vi "rsscope_core_global.vi"() -> ()   [LabVIEW 2018] (continued)
the advanced jitter measurement subsystem (option K133). You can set a separate scale for the symbol rate and symbol duration basic jitter components. You can also set one scale for all other jitter components."}, {"Level"=6, "Class Only"=FALSE, "Identifier"="RSSCOPE_ATTR_ADVANCED_JITTER_RESULTS_SCALING_MAX_NUM_OF_BINS", "Descriptive Name"="Advanced Jitter Results Scaling Max Num Of Bins", "Data Type"=0, "Command"="ADVJ{AdvJitterMeas}:RES:VERT:HBIN", "Access"=2, "Range Table"="RsScope_rngAdvancedJitterHistogramBins", "Read Callback"="", "Write Callback"="", "Supported Models"="", "Instrument Options"="K133|K134", "Flags"=0, "Help"="Sets the number of bins, the number of data intervals, of the histogram.\n\nAvailable Repeated Capabilities:\nAdvJitterMeas: JA1, JA2\r\n\nRemote-control command(s):\nADVJitter<m>:RESult:VERTical:HBINs"}, {"Level"=6, "Class Only"=FALSE, "Identifier"="RSSCOPE_ATTR_ADVANCED_JITTER_RESULTS_CONTINUOUS_AUTO_SCALE_ENABLED", "Descriptive Name"="Advanced Jitter Results Continuous Auto Scale Enabled", "Data Type"=3, "Command"="ADVJ{AdvJitterMeas}:RES:VERT:CONT", "Access"=2, "Range Table"="", "Read Callback"="", "Write Callback"="", "Supported Models"="", "Instrument Options"="K133|K134", "Flags"=0, "Help"="If enabled, the measurement scale is set automatically. If disabled you can manually set a RSSCOPE_ATTR_ADVANCED_JITTER_RESULTS_COMPONENT_SCALE and a RSSCOPE_ATTR_ADVANCED_JITTER_RESULTS_COMPONENT_OFFSET.\n\nAvailable Repeated Capabilities:\nAdvJitterMeas: JA1, JA2\r\n\nRemote-control command(s):\nADVJitter<m>:RESult:VERTical:CONTinuous"}, {"Level"=6, "Class Only"=FALSE, "Identifier"="RSSCOPE_ATTR_ADVANCED_JITTER_RESULTS_BASIC_JITTER_CONTINUOUS_AUTO_SCALE_ENABLED", "Descriptive Name"="Advanced Jitter Results Basic Jitter Continuous Auto Scale Enabled", "Data Type"=3, "Command"="ADVJ{AdvJitterMeas}:RES:VERT:BHC", "Access"=2, "Range Table"="", "Read Callback"="", "Write Callback"="", "Supported Models"="", "Instrument Options"="K133|K134", "Flags"=0, "Help"="If enabled, the measurement scale of the basic jitter measurement histogram and track is set automatically. If disabled you can manually set a scale (RSSCOPE_ATTR_ADVANCED_JITTER_RESULTS_COMPONENT_SCALE) and an offset (RSSCOPE_ATTR_ADVANCED_JITTER_RESULTS_COMPONENT_OFFSET).\n\nAvailable Repeated Capabilities:\nAdvJitterMeas: JA1, JA2\r\n\nRemote-control command(s):\nADVJitter<m>:RESult:VERTical:BHContinuous"}, {"Level"=6, "Class Only"=FALSE, "Identifier"="RSSCOPE_ATTR_ADVANCED_JITTER_RESULTS_NOISE_CONTINUOUS_AUTO_SCALE_ENABLED", "Descriptive Name"="Advanced Jitter Results Noise Continuous Auto Scale Enabled", "Data Type"=3, "Command"="ADVJ{AdvJitterMeas}:RES:VERT:NHC", "Access"=2, "Range Table"="", "Read Callback"="", "Write Callback"="", "Supported Models"="", "Instrument Options"="K133|K134", "Flags"=0, "Help"="If enabled, the measurement scale of the noise histogram and track is set automatically. If disabled you can manually set a scale (RSSCOPE_ATTR_ADVANCED_JITTER_RESULTS_COMPONENT_SCALE) and an offset (RSSCOPE_ATTR_ADVANCED_JITTER_RESULTS_COMPONENT_OFFSET).\n\nAvailable Repeated Capabilities:\nAdvJitterMeas: JA1, JA2\r\n\nRemote-control command(s):\nADVJitter<m>:RESult:VERTical:NHContinuous"}, {"Level"=6, "Class Only"=FALSE, "Identifier"="RSSCOPE_ATTR_ADVANCED_JITTER_RESULTS_JITTER_SPECTRUM_CONTINUOUS_AUTO_SCALE_ENABLED", "Descriptive Name"="Advanced Jitter Results Jitter Spectrum Continuous Auto Scale Enabled", "Data Type"=3, "Command"="ADVJ{AdvJitterMeas}:RES:VERT:JSC", "Access"=2, "Range Table"="", "Read Callback"="", "Write Callback"="", "Supported Models"="", "Instrument Options"="K133|K134", "Flags"=0, "Help"="If enabled, the measurement scale of the jitter spectrum is set automatically. If disabled you can manually set a scale (RSSCOPE_ATTR_ADVANCED_JITTER_RESULTS_COMPONENT_SCALE) and an offset (RSSCOPE_ATTR_ADVANCED_JITTER_RESULTS_COMPONENT_OFFSET).\n\nAvailable Repeated Capabilities:\nAdvJitterMeas: JA1, JA2\r\n\nRemote-control command(s):\nADVJitter<m>:RESult:VERTical:JSContinuous"}, {"Level"=6, "Class Only"=FALSE, "Identifier"="RSSCOPE_ATTR_ADVANCED_JITTER_RESULTS_NOISE_SPECTRUM_CONTINUOUS_AUTO_SCALE_ENABLED", "Descriptive Name"="Advanced Jitter Results Noise Spectrum Continuous Auto Scale Enabled", "Data Type"=3, "Command"="ADVJ{AdvJitterMeas}:RES:VERT:NSC", "Access"=2, "Range Table"="", "Read Callback"="", "Write Callback"="", "Supported Models"="", "Instrument Options"="K133|K134", "Flags"=0, "Help"="If enabled, the measurement scale for the noise spectrum is set automatically. If disabled you can manually set a scale (RSSCOPE_ATTR_ADVANCED_JITTER_RESULTS_COMPONENT_SCALE) and an offset (RSSCOPE_ATTR_ADVANCED_JITTER_RESULTS_COMPONENT_OFFSET).\n\nAvailable Repeated Capabilities:\nAdvJitterMeas: JA1, JA2\r\n\nRemote-control command(s):\nADVJitter<m>:RESult:VERTical:NSContinuous"}, {"Level"=6, "Class Only"=FALSE, "Identifier"="RSSCOPE_ATTR_ADVANCED_JITTER_RESULTS_SCALING_MEASUREMENT_TYPE", "Descriptive Name"="Advanced Jitter Results Scaling Measurement Type", "Data Type"=0, "Command"="ADVJ{AdvJitterMeas}:RES:VERT:BMTY", "Access"=2, "Range Table"="RsScope_rngAdvancedJitterScalingMeasurement", "Read Callback"="", "Write Callback"="", "Supported Models"="", "Instrument Options"="K133|K134", "Flags"=0, "Help"="Selects the basic measurement type to apply the vertical scale to.\n\nAvailable Repeated Capabilities:\nAdvJitterMeas: JA1, JA2\r\n\nRemote-control command(s):\nADVJitter<m>:RESult:VERTical:BMTYpe"}, {"Level"=5, "Class Only"=TRUE, "Identifier"="", "Descriptive Name"="Periodic", "Data Type"=0, "Command"="", "Access"=0, "Range Table"="", "Read Callback"="", "Write Callback"="", "Supported Models"="", "Instrument Options"="", "Flags"=0, "Help"="This class contains results specific to periodic components in the advanced jitter measurement subsystem (option K133)"}, {"Level"=6, "Class Only"=FALSE, "Identifier"="RSSCOPE_ATTR_ADVANCED_JITTER_RESULTS_PERIODIC_COMPONENT_COUNT", "Descriptive Name"="Advanced Jitter Results Periodic Component Count", "Data Type"=0, "Command"="ADVJ{AdvJitterMeas}:RES:PER:COUN?", "Access"=0, "Range Table"="", "Read Callback"="", "Write Callback"="", "Supported Models"="", "Instrument Options"="K133|K134", "Flags"=0, "Help"="Returns the number of periodic components.\n\nAvailable Repeated Capabilities:\nAdvJitterMeas: JA1, JA2\r\n\nRemote-control command(s):\nADVJitter<m>:RESult:PERiodic<n>:COUNt?"}, {"Level"=6, "Class Only"=FALSE, "Identifier"="RSSCOPE_ATTR_ADVANCED_JITTER_RESULTS_PERIODIC_COMPONENT_FREQUENCY", "Descriptive Name"="Advanced Jitter Results Periodic Component Frequency", "Data Type"=5, "Command"="ADVJ{AdvJitterMeas}:RES:PER{AdvJitterPeriodicComponent}?", "Access"=0, "Range Table"="RsScope_rngAdvancedJitterPeriodicFrequency", "Read Callback"="", "Write Callback"="", "Supported Models"="", "Instrument Options"="K133|K134", "Flags"=0, "Help"="Returns the frequency of the selected periodic component.\n\nAvailable Repeated Capabilities:\nAdvJitterMeas: JA1, JA2\r\nAdvJitterPeriodicComponent: Periodic1, Periodic2, Periodic3, Periodic4, Periodic5, Periodic6, Periodic7, Periodic8, Periodic9, Periodic10\r\n\nRemote-control command(s):\nADVJitter<m>:RESult:PERiodic<n>[:FREQuency]?"}, {"Level"=6, "Class Only"=FALSE, "Identifier"="RSSCOPE_ATTR_ADVANCED_JITTER_RESULTS_PERIODIC_COMPONENT_VALUE", "Descriptive Name"="Advanced Jitter Results Periodic Component Value", "Data Type"=1, "Command"="ADVJ{AdvJitterMeas}:RES:PER{AdvJitterPeriodicComponent}:VAL?", "Access"=0, "Range Table"="", "Read Callback"="", "Write Callback"="", "Supported Models"="", "Instrument Options"="K133|K134", "Flags"=0, "Help"="Returns the value of the selected periodic component.\n\nAvailable Repeated Capabilities:\nAdvJitterMeas: JA1, JA2\r\nAdvJitterPeriodicComponent: Periodic1, Periodic2, Periodic3, Periodic4, Periodic5, Periodic6, Periodic7, Periodic8, Periodic9, Periodic10\r\n\nRemote-control command(s):\nADVJitter<m>:RESult:PERiodic<n>:VALue?"}, {"Level"=6, "Class Only"=FALSE, "Identifier"="RSSCOPE_ATTR_ADVANCED_JITTER_RESULTS_PERIODIC_COMPONENT_DIRECTION", "Descriptive Name"="Advanced Jitter Results Periodic Component Direction", "Data Type"=0, "Command"="ADVJ{AdvJitterMeas}:RES:PER{AdvJitterPeriodicComponent}:DIR?", "Access"=0, "Range Table"="RsScope_rngAdvancedJitterPeriodicDirection", "Read Callback"="", "Write Callback"="", "Supported Models"="", "Instrument Options"="K133|K134", "Flags"=0, "Help"="Returns the direction of the selected periodic component.\n\nAvailable Repeated Capabilities:\nAdvJitterMeas: JA1, JA2\r\nAdvJitterPeriodicComponent: Periodic1, Periodic2, Periodic3, Periodic4, Periodic5, Periodic6, Periodic7, Periodic8, Periodic9, Periodic10\r\n\nRemote-control command(s):\nADVJitter<m>:RESult:PERiodic<n>:DIRection?"}, {"Level"=2, "Class Only"=TRUE, "Identifier"="", "Descriptive Name"="Eye Jitter Measurements", "Data Type"=0, "Command"="", "Access"=0, "Range Table"="", "Read Callback"="", "Write Callback"="", "Supported Models"="", "Instrument Options"="", "Flags"=0, "Help"="The eye diagram is a significant means of visualizing jitter and allows you to analyze the reasons for it. Characteristic values can be identified in the eye diagram, and by creating histograms of the eye diagram, important jitter parameters can be determined. In the R&S RTO, the eye diagram is automatically set up for jitter measurements."}, {"Level"=3, "Class Only"=FALSE, "Identifier"="RSSCOPE_ATTR_EYE_MAIN_MEASUREMENT", "Descriptive Name"="Eye Jitter Main Measurement", "Data Type"=0, "Command"="MEAS{Measurement}:MAIN", "Access"=2, "Range Table"="rsscope_rngEyeJitterMeasurementType", "Read Callback"="", "Write Callback"="", "Supported Models"="", "Instrument Options"="", "Flags"=0, "Help"="Defines or queries the main measurement. This measurement is the one referred to if the measurement waveform is used as a source for math calculations. The main measurement type must belong to the same category as the other types assigned to the same measurement waveform, if there are any.\n\nAvailable Repeated Capabilities:\nMeasurement: Meas1, Meas2, Meas3, Meas4, Meas5, Meas6, Meas7, Meas8, Meas9, Meas10\r\n\nRemote-control command(s):\nMEASurement<m>:MAIN"}, {"Level"=3, "Class Only"=FALSE, "Identifier"="RSSCOPE_ATTR_EYE_JITTER_AUTOSCALE", "Descriptive Name"="Eye Jitter Autoscale", "Data Type"=4, "Command"="MEAS{Measurement}:EYEJ:AUT", "Access"=1, "Range Table"="", "Read Callback"="", "Write Callback"="", "Supported Models"="", "Instrument Options"="", "Flags"=0, "Help"="Defines optimized settings to perform an eye diagram measurement for the selected source.\n\nAvailable Repeated Capabilities:\nMeasurement: Meas1, Meas2, Meas3, Meas4, Meas5, Meas6, Meas7, Meas8, Meas9, Meas10\r\n\nRemote-control command(s):\nMEASurement<m>:EYEJitter:AUToscale"}, {"Level"=3, "Class Only"=TRUE, "Identifier"="", "Descriptive Name"="Eye Measurement Type", "Data Type"=0, "Command"="", "Access"=0, "Range Table"="", "Read Callback"="", "Write Callback"="", "Supported Models"="", "Instrument Options"="", "Flags"=0, "Help"="Selects Eye Measurement Type"}, {"Level"=4, "Class Only"=FALSE, "Identifier"="RSSCOPE_ATTR_EYE_LIMIT_CHECK", "Descriptive Name"="Eye Jitter Limit Check", "Data Type"=0, "Command"="MEAS{Measurement}:EYEJ:LCH{EyeMeasurementType}:VAL", "Access"=2, "Range Table"="rsscope_rngLimitCheck", "Read Callback"="", "Write Callback"="", "Supported Models"="", "Instrument Options"="", "Flags"=0, "Help"="Enables or disables limit checking for eye/jitter measurements in the specified measurement channel.\n\nAvailable Repeated Capabilities:\nMeasurement: Meas1, Meas2, Meas3, Meas4, Meas5, Meas6, Meas7, Meas8, Meas9, Meas10\r\nEyeMeasurementType: Eye1, Eye2, Eye3, Eye4, Eye5, Eye6, Eye7, Eye8, Eye9, Eye10, Eye11, Eye12, Eye13, Eye14, Eye15, Eye16, Eye17, Eye18, Eye19, Eye20, Eye21, Eye22, Eye23, Eye24, Eye25, Eye26, Eye27, Eye28, Eye29, Eye30\r\n\nRemote-control command(s):\nMEASurement<m>:EYEJitter:LCHeck<n>:VALid"}, {"Level"=4, "Class Only"=FALSE, "Identifier"="RSSCOPE_ATTR_EYE_JITTER_LOWER_LIMIT_VALUE", "Descriptive Name"="Eye Jitter Lower Limit Value", "Data Type"=1, "Command"="MEAS{Measurement}:EYEJ:LCH{EyeMeasurementType}:LOW:LIM", "Access"=2, "Range Table"="", "Read Callback"="", "Write Callback"="", "Supported Models"="", "Instrument Options"="", "Flags"=0, "Help"="Define the lower limit for the limit check.\n\nAvailable Repeated Capabilities:\nMeasurement: Meas1, Meas2, Meas3, Meas4, Meas5, Meas6, Meas7, Meas8, Meas9, Meas10\r\nEyeMeasurementType: Eye1, Eye2, Eye3, Eye4, Eye5, Eye6, Eye7, Eye8, Eye9, Eye10, Eye11, Eye12, Eye13, Eye14, Eye15, Eye16, Eye17, Eye18, Eye19, Eye20, Eye21, Eye22, Eye23, Eye24, Eye25, Eye26, Eye27, Eye28, Eye29, Eye30\r\n\nRemote-control command(s):\nMEASurement<m>:EYEJitter:LCHeck<n>:LOWer:LIMit"}, {"Level"=4, "Class Only"=FALSE, "Identifier"="RSSCOPE_ATTR_EYE_JITTER_UPPER_LIMIT_VALUE", "Descriptive Name"="Eye Jitter Upper Limit Value", "Data Type"=1, "Command"="MEAS{Measurement}:EYEJ:LCH{EyeMeasurementType}:UPP:LIM", "Access"=2, "Range Table"="", "Read Callback"="", "Write Callback"="", "Supported Models"="", "Instrument Options"="", "Flags"=0, "Help"="Define the upper limit for the limit check.\n\nAvailable Repeated Capabilities:\nMeasurement: Meas1, Meas2, Meas3, Meas4, Meas5, Meas6, Meas7, Meas8, Meas9, Meas10\r\nEyeMeasurementType: Eye1, Eye2, Eye3, Eye4, Eye5, Eye6, Eye7, Eye8, Eye9, Eye10, Eye11, Eye12, Eye13, Eye14, Eye15, Eye16, Eye17, Eye18, Eye19, Eye20, Eye21, Eye22, Eye23, Eye24, Eye25, Eye26, Eye27, Eye28, Eye29, Eye30\r\n\nRemote-control command(s):\nMEASurement<m>:EYEJitter:LCHeck<n>:UPPer:LIMit"}, {"Level"=4, "Class Only"=FALSE, "Identifier"="RSSCOPE_ATTR_EYE_JITTER_LOWER_LIMIT_MARGIN", "Descriptive Name"="Eye Jitter Lower Limit Margin", "Data Type"=1, "Command"="MEAS{Measurement}:EYEJ:LCH{EyeMeasurementType}:LOW:MARG", "Access"=2, "Range Table"="", "Read Callback"="", "Write Callback"="", "Supported Models"="", "Instrument Options"="", "Flags"=0, "Help"="Defines the lower margin for the limit check. Margins are not as strict as limits and must be within the valid value range.\n\nAvailable Repeated Capabilities:\nMeasurement: Meas1, Meas2, Meas3, Meas4, Meas5, Meas6, Meas7, Meas8, Meas9, Meas10\r\nEyeMeasurementType: Eye1, Eye2, Eye3, Eye4, Eye5, Eye6, Eye7, Eye8, Eye9, Eye10, Eye11, Eye12, Eye13, Eye14, Eye15, Eye16, Eye17, Eye18, Eye19, Eye20, Eye21, Eye22, Eye23, Eye24, Eye25, Eye26, Eye27, Eye28, Eye29, Eye30\r\n\nRemote-control command(s):\nMEASurement<m>:EYEJitter:LCHeck<n>:LOWer:MARGin"}, {"Level"=4, "Class Only"=FALSE, "Identifier"="RSSCOPE_ATTR_EYE_JITTER_UPPER_LIMIT_MARGIN", "Descriptive Name"="Eye Jitter Upper Limit Margin", "Data Type"=1, "Command"="MEAS{Measurement}:EYEJ:LCH{EyeMeasurementType}:UPP:MARG", "Access"=2, "Range Table"="", "Read Callback"="", "Write Callback"="", "Supported Models"="", "Instrument Options"="", "Flags"=0, "Help"="Defines the upper margin for the limit check. Margins are not as strict as limits and must be within the valid value range.\n\nAvailable Repeated Capabilities:\nMeasurement: Meas1, Meas2, Meas3, Meas4, Meas5, Meas6, Meas7, Meas8, Meas9, Meas10\r\nEyeMeasurementType: Eye1, Eye2, Eye3, Eye4, Eye5, Eye6, Eye7, Eye8, Eye9, Eye10, Eye11, Eye12, Eye13, Eye14, Eye15, Eye16, Eye17, Eye18, Eye19, Eye20, Eye21, Eye22, Eye23, Eye24, Eye25, Eye26, Eye27, Eye28, Eye29, Eye30\r\n\nRemote-control command(s):\nMEASurement<m>:EYEJitter:LCHeck<n>:UPPer:MARGin"}, {"Level"=2, "Class Only"=TRUE, "Identifier"="", "Descriptive Name"="Histograms", "Data Type"=0, "Command"="", "Access"=0, "Range Table"="", "Read Callback"="", "Write Callback"="", "Supported Models"="", "Instrument Options"="", "Flags"=0, "Help"="Histograms are used to plot density of data, i.e. to display graphically how often which signal values occur. In the R&S RTO, the histogram can be based on the input signal levels (amplitudes) or the time base in a time domain measurement, or on frequencies or frequency levels in a spectrum measurement.\nDepending on which data the histogram is based on, a vertical or horizontal histogram can be selected. A vertical, or amplitude, histogram displays horizontal bars across amplitude values. A horizontal or time/frequency histogram displays vertical bars over time/frequencies."}, {"Level"=3, "Class Only"=FALSE, "Identifier"="RSSCOPE_ATTR_HISTOGRAM_MAIN_MEASUREMENT", "Descriptive Name"="Histogram Main Measurement", "Data Type"=0, "Command"="MEAS{Measurement}:MAIN", "Access"=2, "Range Table"="rsscope_rngHistogramMeasurementType", "Read Callback"="", "Write Callback"="", "Supported Models"="", "Instrument Options"="", "Flags"=0, "Help"="Defines or queries the main measurement. This measurement is the one referred to if the measurement waveform is used as a source for math calculations. The main measurement type must belong to the same category as the other types assigned to the same measurement waveform, if there are any.\n\nAvailable Repeated Capabilities:\nMeasurement: Meas1, Meas2, Meas3, Meas4, Meas5, Meas6, Meas7, Meas8, Meas9, Meas10\r\n\nRemote-control command(s):\nMEASurement<m>:MAIN"}, {"Level"=3, "Class Only"=FALSE, "Identifier"="RSSCOPE_ATTR_HISTOGRAM_SELECT", "Descriptive Name"="Histogram Select", "Data Type"=2, "Command"="MEAS{Measurement}:HIST:SEL", "Access"=2, "Range Table"="", "Read Callback"="", "Write Callback"="", "Supported Models"="", "Instrument Options"="", "Flags"=0, "Help"="Selects the histogram on which the measurement is based.\n\nAvailable Repeated Capabilities:\nMeasurement: Meas1, Meas2, Meas3, Meas4, Meas5, Meas6, Meas7, Meas8, Meas9, Meas10\r\n\nRemote-control command(s):\nMEASurement<m>:HISTogram:SELect"}, {"Level"=3, "Class Only"=FALSE, "Identifier"="RSSCOPE_ATTR_HISTOGRAM_PROBABILITY_TYPE", "Descriptive Name"="Histogram Probability Type", "Data Type"=0, "Command"="MEAS{Measurement}:HIST:PROB:TYPE", "Access"=2, "Range Table"="rsscope_rngProbabilityType", "Read Callback"="", "Write Callback"="", "Supported Models"="", "Instrument Options"="", "Flags"=0, "Help"="Defines the marker reference in the probability domain.\n\nAvailable Repeated Capabilities:\nMeasurement: Meas1, Meas2, Meas3, Meas4, Meas5, Meas6, Meas7, Meas8, Meas9, Meas10\r\n\nRemote-control command(s):\nMEASurement<m>:HISTogram:PROBability:TYPE"}, {"Level"=3, "Class Only"=FALSE, "Identifier"="RSSCOPE_ATTR_HISTOGRAM_PROBABILITY_LIMIT", "Descriptive Name"="Histogram Probability Limit", "Data Type"=0, "Command"="MEAS{Measurement}:HIST:PROB:LIM", "Access"=2, "Range Table"="rsscope_rngPct", "Read Callback"="", "Write Callback"="", "Supported Models"="", "Instrument Options"="", "Flags"=0, "Help"="Defines a range around the probability marker.\n\nAvailable Repeated Capabilities:\nMeasurement: Meas1, Meas2, Meas3, Meas4, Meas5, Meas6, Meas7, Meas8, Meas9, Meas10\r\n\nRemote-control command(s):\nMEASurement<m>:HISTogram:PROBability:LIMit"}, {"Level"=3, "Class Only"=FALSE, "Identifier"="RSSCOPE_ATTR_REMOVE_HISTOGRAM", "Descriptive Name"="Remove Histogram", "Data Type"=2, "Command"="LAY:HIST:REM", "Access"=1, "Range Table"="", "Read Callback"="", "Write Callback"="", "Supported Models"="", "Instrument Options"="", "Flags"=0, "Help"="Removes the specified histogram.\n\nAvailable Repeated Capabilities:\nNone\n\nRemote-control command(s):\nLAYout:HISTogram:REMove"}, {"Level"=3, "Class Only"=FALSE, "Identifier"="RSSCOPE_ATTR_RESET_HISTOGRAM", "Descriptive Name"="Reset Histogram", "Data Type"=2, "Command"="LAY:HIST:RES", "Access"=1, "Range Table"="", "Read Callback"="", "Write Callback"="", "Supported Models"="", "Instrument Options"="", "Flags"=0, "Help"="Resets the values to begin a new histogram.\n\nAvailable Repeated Capabilities:\nNone\n\nRemote-control command(s):\nLAYout:HISTogram:RESet"}, {"Level"=3, "Class Only"=FALSE, "Identifier"="RSSCOPE_ATTR_HISTOGRAM_DISPLAY", "Descriptive Name"="Histogram Display", "Data Type"=3, "Command"="MEAS{Measurement}:DISP:HIST", "Access"=2, "Range Table"="", "Read Callback"="", "Write Callback"="", "Supported Models"="", "Instrument Options"="", "Flags"=0, "Help"="Displays a histogram for the source of the selected measurement.\n\nAvailable Repeated Capabilities:\nMeasurement: Meas1, Meas2, Meas3, Meas4, Meas5, Meas6, Meas7, Meas8, Meas9, Meas10\r\n\nRemote-control command(s):\nMEASurement<m>:DISPlay:HISTogram"}, {"Level"=3, "Class Only"=TRUE, "Identifier"="", "Descriptive Name"="Histogram Measurement Type", "Data Type"=0, "Command"="", "Access"=0, "Range Table"="", "Read Callback"="", "Write Callback"="", "Supported Models"="", "Instrument Options"="", "Flags"=0, "Help"="Selects Histogram Measurement Type"}, {"Level"=4, "Class Only"=FALSE, "Identifier"="RSSCOPE_ATTR_HISTOGRAM_LIMIT_CHECK", "Descriptive Name"="Histogram Limit Check", "Data Type"=0, "Command"="MEAS{Measurement}:HIST:LCH{HistogramMeasurementType}:VAL", "Access"=2, "Range Table"="rsscope_rngLimitCheck", "Read Callback"="", "Write Callback"="", "Supported Models"="", "Instrument Options"="", "Flags"=0, "Help"="Enables or disables limit checking for histogram measurements in the specified measurement channel.\n\nAvailable Repeated Capabilities:\nMeasurement: Meas1, Meas2, Meas3, Meas4, Meas5, Meas6, Meas7, Meas8, Meas9, Meas10\r\nHistogramMeasurementType: Hist1, Hist2, Hist3, Hist4, Hist5, Hist6, Hist7, Hist8, Hist9, Hist10, Hist11, Hist12, Hist13, Hist14, Hist15, Hist16, Hist17, Hist18\r\n\nRemote-control command(s):\nMEASurement<m>:HISTogram:LCHeck<n>:VALid"}, {"Level"=4, "Class Only"=FALSE, "Identifier"="RSSCOPE_ATTR_HISTOGRAM_LOWER_LIMIT_VALUE", "Descriptive Name"="Histogram Lower Limit Value", "Data Type"=1, "Command"="MEAS{Measurement}:HIST:LCH{HistogramMeasurementType}:LOW:LIM", "Access"=2, "Range Table"="", "Read Callback"="", "Write Callback"="", "Supported Models"="", "Instrument Options"="", "Flags"=0, "Help"="Define the lower limit for the limit check.\n\nAvailable Repeated Capabilities:\nMeasurement: Meas1, Meas2, Meas3, Meas4, Meas5, Meas6, Meas7, Meas8, Meas9, Meas10\r\nHistogramMeasurementType: Hist1, Hist2, Hist3, Hist4, Hist5, Hist6, Hist7, Hist8, Hist9, Hist10, Hist11, Hist12, Hist13, Hist14, Hist15, Hist16, Hist17, Hist18\r\n\nRemote-control command(s):\nMEASurement<m>:HISTogram:LCHeck<n>:LOWer:LIMit"}, {"Level"=4, "Class Only"=FALSE, "Identifier"="RSSCOPE_ATTR_HISTOGRAM_UPPER_LIMIT_VALUE", "Descriptive Name"="Histogram Upper Limit Value", "Data Type"=1, "Command"="MEAS{Measurement}:HIST:LCH{HistogramMeasurementType}:UPP:LIM", "Access"=2, "Range Table"="", "Read Callback"="", "Write Callback"="", "Supported Models"="", "Instrument Options"="", "Flags"=0, "Help"="Define the upper limit for the limit check.\n\nAvailable Repeated Capabilities:\nMeasurement: Meas1, Meas2, Meas3, Meas4, Meas5, Meas6, Meas7, Meas8, Meas9, Meas10\r\nHistogramMeasurementType: Hist1, Hist2, Hist3, Hist4, Hist5, Hist6, Hist7, Hist8, Hist9, Hist10, Hist11, Hist12, Hist13, Hist14, Hist15, Hist16, Hist17, Hist18\r\n\nRemote-control command(s):\nMEASurement<m>:HISTogram:LCHeck<n>:UPPer:LIMit"}, {"Level"=4, "Class Only"=FALSE, "Identifier"="RSSCOPE_ATTR_HISTOGRAM_LOWER_LIMIT_MARGIN", "Descriptive Name"="Histogram Lower Limit Margin", "Data Type"=1, "Command"="MEAS{Measurement}:HIST:LCH{HistogramMeasurementType}:LOW:MARG", "Access"=2, "Range Table"="", "Read Callback"="", "Write Callback"="", "Supported Models"="", "Instrument Options"="", "Flags"=0, "Help"="Define the lower margin for the limit check. Margins are not as strict as limits and must be within the valid value range.\n\nAvailable Repeated Capabilities:\nMeasurement: Meas1, Meas2, Meas3, Meas4, Meas5, Meas6, Meas7, Meas8, Meas9, Meas10\r\nHistogramMeasurementType: Hist1, Hist2, Hist3, Hist4, Hist5, Hist6, Hist7, Hist8, Hist9, Hist10, Hist11, Hist12, Hist13, Hist14, Hist15, Hist16, Hist17, Hist18\r\n\nRemote-control command(s):\nMEASurement<m>:HISTogram:LCHeck<n>:LOWer:MARGin"}, {"Level"=4, "Class Only"=FALSE, "Identifier"="RSSCOPE_ATTR_HISTOGRAM_UPPER_LIMIT_MARGIN", "Descriptive Name"="Histogram Upper Limit Margin", "Data Type"=1, "Command"="MEAS{Measurement}:HIST:LCH{HistogramMeasurementType}:UPP:MARG", "Access"=2, "Range Table"="", "Read Callback"="", "Write Callback"="", "Supported Models"="", "Instrument Options"="", "Flags"=0, "Help"="Define the upper margins for the limit check. Margins are not as strict as limits and must be within the valid value range.\n\nAvailable Repeated Capabilities:\nMeasurement: Meas1, Meas2, Meas3, Meas4, Meas5, Meas6, Meas7, Meas8, Meas9, Meas10\r\nHistogramMeasurementType: Hist1, Hist2, Hist3, Hist4, Hist5, Hist6, Hist7, Hist8, Hist9, Hist10, Hist11, Hist12, Hist13, Hist14, Hist15, Hist16, Hist17, Hist18\r\n\nRemote-control command(s):\nMEASurement<m>:HISTogram:LCHeck<n>:UPPer:MARGin"}, {"Level"=2, "Class Only"=TRUE, "Identifier"="", "Descriptive Name"="Spectrum Measurements", "Data Type"=0, "Command"="", "Access"=0, "Range Table"="", "Read Callback"="", "Write Callback"="", "Supported Models"="", "Instrument Options"="", "Flags"=0, "Help"="Spectrum analysis determines the frequencies of a given input signal over time. Various measurements can then be performed based on the signal spectrum."}, {"Level"=3, "Class Only"=FALSE, "Identifier"="RSSCOPE_ATTR_SPECTRUM_MAIN_MEASUREMENT", "Descriptive Name"="Spectrum Main Measurement", "Data Type"=0, "Command"="MEAS{Measurement}:MAIN", "Access"=2, "Range Table"="rsscope_rngSpectrumMeasurementType", "Read Callback"="", "Write Callback"="", "Supported Models"="", "Instrument Options"="", "Flags"=0, "Help"="Defines or queries the main measurement. This measurement is the one referred to if the measurement waveform is used as a source for math calculations. The main measurement type must belong to the same category as the other types assigned to the same measurement waveform, if there are any.\n\nAvailable Repeated Capabilities:\nMeasurement: Meas1, Meas2, Meas3, Meas4, Meas5, Meas6, Meas7, Meas8, Meas9, Meas10\r\n\nRemote-control command(s):\nMEASurement<m>:MAIN"}, {"Level"=3, "Class Only"=FALSE, "Identifier"="RSSCOPE_ATTR_SPECTRUM_CHANNEL_POWER_BANDWIDTH", "Descriptive Name"="Spectrum Channel Power Bandwidth", "Data Type"=1, "Command"="MEAS{Measurement}:SPEC:CPOW:BAND", "Access"=2, "Range Table"="RsScope_rngSCBandwidth", "Read Callback"="", "Write Callback"="", "Supported Models"="", "Instrument Options"="", "Flags"=0, "Help"="Defines the bandwidth over which the channel power is calculated.\n\nAvailable Repeated Capabilities:\nMeasurement: Meas1, Meas2, Meas3, Meas4, Meas5, Meas6, Meas7, Meas8, Meas9, Meas10\r\n\nRemote-control command(s):\nMEASurement<m>:SPECtrum:CPOWer:BANDwidth"}, {"Level"=3, "Class Only"=FALSE, "Identifier"="RSSCOPE_ATTR_SPECTRUM_OCCUPIED_BANDWIDTH", "Descriptive Name"="Spectrum Occupied Bandwidth", "Data Type"=1, "Command"="MEAS{Measurement}:SPEC:OBAN", "Access"=2, "Range Table"="rsscope_rngObw", "Read Callback"="", "Write Callback"="", "Supported Models"="", "Instrument Options"="", "Flags"=0, "Help"="Defines the percentage of the total power used to determine the occupied bandwidth.\n\nAvailable Repeated Capabilities:\nMeasurement: Meas1, Meas2, Meas3, Meas4, Meas5, Meas6, Meas7, Meas8, Meas9, Meas10\r\n\nRemote-control command(s):\nMEASurement<m>:SPECtrum:OBANdwidth"}, {"Level"=3, "Class Only"=FALSE, "Identifier"="RSSCOPE_ATTR_SPECTRUM_CHANNEL_POWER_CENTER_FREQUENCY", "Descriptive Name"="Spectrum Channel Power Center Frequency", "Data Type"=1, "Command"="MEAS{Measurement}:SPEC:CPOW:CFR", "Access"=2, "Range Table"="rsscope_rngBandwidth", "Read Callback"="", "Write Callback"="", "Supported Models"="", "Instrument Options"="", "Flags"=0, "Help"="Defines the center frequency from which the channel power is calculated over the specified bandwidth.\n\nAvailable Repeated Capabilities:\nMeasurement: Meas1, Meas2, Meas3, Meas4, Meas5, Meas6, Meas7, Meas8, Meas9, Meas10\r\n\nRemote-control command(s):\nMEASurement<m>:SPECtrum:CPOWer:CFRequency"}, {"Level"=3, "Class Only"=FALSE, "Identifier"="RSSCOPE_ATTR_SPECTRUM_N_DB_DOWN", "Descriptive Name"="Spectrum n dB Down", "Data Type"=0, "Command"="MEAS{Measurement}:SPEC:NDBD", "Access"=2, "Range Table"="rsscope_rngPct", "Read Callback"="", "Write Callback"="", "Supported Models"="", "Instrument Options"="", "Flags"=0, "Help"="Defines the threshold until which the samples to the left and right of the peak value are analyzed in order to determine the &apos;N dB down bandwidth&apos;.\n\nAvailable Repeated Capabilities:\nMeasurement: Meas1, Meas2, Meas3, Meas4, Meas5, Meas6, Meas7, Meas8, Meas9, Meas10\r\n\nRemote-control command(s):\nMEASurement<m>:SPECtrum:NDBDown"}, {"Level"=3, "Class Only"=FALSE, "Identifier"="RSSCOPE_ATTR_SPECTRUM_PEAK_EXCURSION", "Descriptive Name"="Spectrum Peak Excursion", "Data Type"=0, "Command"="MEAS{Measurement}:SPEC:PEXC", "Access"=2, "Range Table"="rsscope_rngPct", "Read Callback"="", "Write Callback"="", "Supported Models"="", "Instrument Options"="", "Flags"=0, "Help"="Defines a relative threshold, the minimum level value by which the waveform must rise or fall to be considered as a peak. To avoid identifying noise peaks, enter a peak excursion value that is higher than the noise levels.\n\nAvailable Repeated Capabilities:\nMeasurement: Meas1, Meas2, Meas3, Meas4, Meas5, Meas6, Meas7, Meas8, Meas9, Meas10\r\n\nRemote-control command(s):\nMEASurement<m>:SPECtrum:PEXCursion"}, {"Level"=3, "Class Only"=FALSE, "Identifier"="RSSCOPE_ATTR_SPECTRUM_ABSOLUTE_THRESHOLD", "Descriptive Name"="Spectrum Absolute Threshold", "Data Type"=1, "Command"="MEAS{Measurement}:SPEC:ATHR", "Access"=2, "Range Table"="", "Read Callback"="", "Write Callback"="", "Supported Models"="", "Instrument Options"="", "Flags"=0, "Help"="Defines an absolute threshold as an additional condition for the peak search. Only peaks that exceed the threshold are detected.\nThis setting is only available for spectrum waveforms. It is valid for cursor measurements, spectrum measurements and peak search.\n\nAvailable Repeated Capabilities:\nMeasurement: Meas1, Meas2, Meas3, Meas4, Meas5, Meas6, Meas7, Meas8, Meas9, Meas10\r\n\nRemote-control command(s):\nMEASurement<m>:SPECtrum:ATHReshold"}, {"Level"=3, "Class Only"=TRUE, "Identifier"="", "Descriptive Name"="Result Labels", "Data Type"=0, "Command"="", "Access"=0, "Range Table"="", "Read Callback"="", "Write Callback"="", "Supported Models"="", "Instrument Options"="", "Flags"=0, "Help"="For peak lists only: a description of each detected peak can be provided using labels in the spectrum diagram."}, {"Level"=3, "Class Only"=TRUE, "Identifier"="", "Descriptive Name"="Spectrum Measurement Type", "Data Type"=0, "Command"="", "Access"=0, "Range Table"="", "Read Callback"="", "Write Callback"="", "Supported Models"="", "Instrument Options"="", "Flags"=0, "Help"="Selects Spectrum Measurement Type"}, {"Level"=4, "Class Only"=FALSE, "Identifier"="RSSCOPE_ATTR_SPECTRUM_LIMIT_CHECK", "Descriptive Name"="Spectrum Limit Check", "Data Type"=0, "Command"="MEAS{Measurement}:SPEC:LCH{SpectrumMeasurementType}:VAL", "Access"=2, "Range Table"="rsscope_rngLimitCheck", "Read Callback"="", "Write Callback"="", "Supported Models"="", "Instrument Options"="", "Flags"=0, "Help"="Enables or disables limit checking for spectrum measurements in the specified measurement channel.\n\nAvailable Repeated Capabilities:\nMeasurement: Meas1, Meas2, Meas3, Meas4, Meas5, Meas6, Meas7, Meas8, Meas9, Meas10\r\nSpectrumMeasurementType: Spec1, Spec2, Spec3, Spec4, Spec5, Spec6, Spec7, Spec8, Spec9, Spec10, Spec11, Spec12\r\n\nRemote-control command(s):\nMEASurement<m>:SPECtrum:LCHeck<n>:VALid"}, {"Level"=4, "Class Only"=FALSE, "Identifier"="RSSCOPE_ATTR_SPECTRUM_LOWER_LIMIT_VALUE", "Descriptive Name"="Spectrum Lower Limit Value", "Data Type"=1, "Command"="MEAS{Measurement}:SPEC:LCH{SpectrumMeasurementType}:LOW:LIM", "Access"=2, "Range Table"="", "Read Callback"="", "Write Callback"="", "Supported Models"="", "Instrument Options"="", "Flags"=0, "Help"="Define the lower limit for the limit check.\n\nAvailable Repeated Capabilities:\nMeasurement: Meas1, Meas2, Meas3, Meas4, Meas5, Meas6, Meas7, Meas8, Meas9, Meas10\r\nSpectrumMeasurementType: Spec1, Spec2, Spec3, Spec4, Spec5, Spec6, Spec7, Spec8, Spec9, Spec10, Spec11, Spec12\r\n\nRemote-control command(s):\nMEASurement<m>:SPECtrum:LCHeck<n>:LOWer:LIMit"}, {"Level"=4, "Class Only"=FALSE, "Identifier"="RSSCOPE_ATTR_SPECTRUM_UPPER_LIMIT_VALUE", "Descriptive Name"="Spectrum Upper Limit Value", "Data Type"=1, "Command"="MEAS{Measurement}:SPEC:LCH{SpectrumMeasurementType}:UPP:LIM", "Access"=2, "Range Table"="", "Read Callback"="", "Write Callback"="", "Supported Models"="", "Instrument Options"="", "Flags"=0, "Help"="Define the upper limit for the limit check.\n\nAvailable Repeated Capabilities:\nMeasurement: Meas1, Meas2, Meas3, Meas4, Meas5, Meas6, Meas7, Meas8, Meas9, Meas10\r\nSpectrumMeasurementType: Spec1, Spec2, Spec3, Spec4, Spec5, Spec6, Spec7, Spec8, Spec9, Spec10, Spec11, Spec12\r\n\nRemote-control command(s):\nMEASurement<m>:SPECtrum:LCHeck<n>:UPPer:LIMit"}, {"Level"=4, "Class Only"=FALSE, "Identifier"="RSSCOPE_ATTR_SPECTRUM_LOWER_LIMIT_MARGIN", "Descriptive Name"="Spectrum Lower Limit Margin", "Data Type"=1, "Command"="MEAS{Measurement}:SPEC:LCH{SpectrumMeasurementType}:LOW:MARG", "Access"=2, "Range Table"="", "Read Callback"="", "Write Callback"="", "Supported Models"="", "Instrument Options"="", "Flags"=0, "Help"="Define the lower margin for the limit check. Margins are not as strict as limits and must be within the valid value range.\n\nAvailable Repeated Capabilities:\nMeasurement: Meas1, Meas2, Meas3, Meas4, Meas5, Meas6, Meas7, Meas8, Meas9, Meas10\r\nSpectrumMeasurementType: Spec1, Spec2, Spec3, Spec4, Spec5, Spec6, Spec7, Spec8, Spec9, Spec10, Spec11, Spec12\r\n\nRemote-control command(s):\nMEASurement<m>:SPECtrum:LCHeck<n>:LOWer:MARGin"}, {"Level"=4, "Class Only"=FALSE, "Identifier"="RSSCOPE_ATTR_SPECTRUM_UPPER_LIMIT_MARGIN", "Descriptive Name"="Spectrum Upper Limit Margin", "Data Type"=1, "Command"="MEAS{Measurement}:SPEC:LCH{SpectrumMeasurementType}:UPP:MARG", "Access"=2, "Range Table"="", "Read Callback"="", "Write Callback"="", "Supported Models"="", "Instrument Options"="", "Flags"=0, "Help"="Define the upper margin for the limit check, respectively. Margins are not as strict as limits and must be within the valid value range.\n\nAvailable Repeated Capabilities:\nMeasurement: Meas1, Meas2, Meas3, Meas4, Meas5, Meas6, Meas7, Meas8, Meas9, Meas10\r\nSpectrumMeasurementType: Spec1, Spec2, Spec3, Spec4, Spec5, Spec6, Spec7, Spec8, Spec9, Spec10, Spec11, Spec12\r\n\nRemote-control command(s):\nMEASurement<m>:SPECtrum:LCHeck<n>:UPPer:MARGin"}, {"Level"=4, "Class Only"=FALSE, "Identifier"="RSSCOPE_ATTR_SPECTRUM_MAX_NUMBER_OF_RESULTS", "Descriptive Name"="Spectrum Max Number Of Results", "Data Type"=0, "Command"="MEAS{Measurement}:SPEC:RES{SpectrumMeasurementType}:COUN", "Access"=2, "Range Table"="RsScope_rngSpectrumMaxNumberOfResults", "Read Callback"="", "Write Callback"="", "Supported Models"="", "Instrument Options"="", "Flags"=0, "Help"="Sets the maximum number of measurement results that are listed in the result table. Available for peak list and harmonic search mesurements.\n\nAvailable Repeated Capabilities:\nMeasurement: Meas1, Meas2, Meas3, Meas4, Meas5, Meas6, Meas7, Meas8, Meas9, Meas10\r\nSpectrumMeasurementType: Spec1, Spec2, Spec3, Spec4, Spec5, Spec6, Spec7, Spec8, Spec9, Spec10, Spec11, Spec12\r\n\nRemote-control command(s):\nMEASurement<m>:SPECtrum:RESult<n>:COUNt"}, {"Level"=4, "Class Only"=FALSE, "Identifier"="RSSCOPE_ATTR_SPECTRUM_RESULT_MODE", "Descriptive Name"="Spectrum Result Mode", "Data Type"=0, "Command"="MEAS{Measurement}:SPEC:RES{SpectrumMeasurementType}:MODE", "Access"=2, "Range Table"="RsScope_rngSpectrumResultMode", "Read Callback"="", "Write Callback"="", "Supported Models"="", "Instrument Options"="", "Flags"=0, "Help"="Sets the way the measurement results are displayed. Available only if RSSCOPE_ATTR_SPECTRUM_MAIN_MEASUREMENT is set to PLISt or HAR.\n\nAvailable Repeated Capabilities:\nMeasurement: Meas1, Meas2, Meas3, Meas4, Meas5, Meas6, Meas7, Meas8, Meas9, Meas10\r\nSpectrumMeasurementType: Spec1, Spec2, Spec3, Spec4, Spec5, Spec6, Spec7, Spec8, Spec9, Spec10, Spec11, Spec12\r\n\nRemote-control command(s):\nMEASurement<m>:SPECtrum:RESult<n>:MODE"}, {"Level"=3, "Class Only"=TRUE, "Identifier"="", "Descriptive Name"="Spectrum Arithmetic", "Data Type"=0, "Command"="", "Access"=0, "Range Table"="", "Read Callback"="", "Write Callback"="", "Supported Models"="", "Instrument Options"="", "Flags"=0, "Help"="Contains attributes to configure the arithmetic for spectrum measurements."}, {"Level"=4, "Class Only"=FALSE, "Identifier"="RSSCOPE_ATTR_SPECTRUM_ARITHMETIC_PARAMETER_MEASUEREMENT_TYPE", "Descriptive Name"="Spectrum Arithmetic Parameter Measuerement Type", "Data Type"=0, "Command"="MEAS{Measurement}:SPEC:ARIT:PAR{ArithmeticParameter}:TYPE", "Access"=2, "Range Table"="RsScope_rngArithmeticMeasurementType", "Read Callback"="", "Write Callback"="", "Supported Models"="", "Instrument Options"="", "Flags"=0, "Help"="Sets the type of spectrum arithmetic measurement.\n\nAvailable Repeated Capabilities:\nMeasurement: Meas1, Meas2, Meas3, Meas4, Meas5, Meas6, Meas7, Meas8, Meas9, Meas10\r\nArithmeticParameter: ArithmeticParm1, ArithmeticParm2\r\n\nRemote-control command(s):\nMEASurement<m>:SPECtrum:ARIThmetic:PARameter<n>:TYPE"}, {"Level"=4, "Class Only"=FALSE, "Identifier"="RSSCOPE_ATTR_SPECTRUM_ARITHMETIC_PARAMETER_AMPLITUDE_TIME", "Descriptive Name"="Spectrum Arithmetic Parameter Amplitude Time", "Data Type"=0, "Command"="MEAS{Measurement}:SPEC:ARIT:PAR{ArithmeticParameter}:AMPT", "Access"=2, "Range Table"="rsscope_rngAmplitudeTimeMeasurementType", "Read Callback"="", "Write Callback"="", "Supported Models"="", "Instrument Options"="", "Flags"=0, "Help"="Selects the amplitude/time arithmetics measurements for the measurment group.\n\nAvailable Repeated Capabilities:\nMeasurement: Meas1, Meas2, Meas3, Meas4, Meas5, Meas6, Meas7, Meas8, Meas9, Meas10\r\nArithmeticParameter: ArithmeticParm1, ArithmeticParm2\r\n\nRemote-control command(s):\nMEASurement<m>:SPECtrum:ARIThmetic:PARameter<n>:AMPTime"}, {"Level"=4, "Class Only"=FALSE, "Identifier"="RSSCOPE_ATTR_SPECTRUM_ARITHMETIC_PARAMETER_GROUP", "Descriptive Name"="Spectrum Arithmetic Parameter Group", "Data Type"=0, "Command"="MEAS{Measurement}:SPEC:ARIT:PAR{ArithmeticParameter}:GRO", "Access"=2, "Range Table"="RsScope_rngSpectrumArithmeticParameterGroup", "Read Callback"="", "Write Callback"="", "Supported Models"="", "Instrument Options"="", "Flags"=0, "Help"="Sets the measurement group for the second operand of the spectrum arithmetic measurement.\n\nAvailable Repeated Capabilities:\nMeasurement: Meas1, Meas2, Meas3, Meas4, Meas5, Meas6, Meas7, Meas8, Meas9, Meas10\r\nArithmeticParameter: ArithmeticParm1, ArithmeticParm2\r\n\nRemote-control command(s):\nMEASurement<m>:SPECtrum:ARIThmetic:PARameter<n>:GROup"}, {"Level"=4, "Class Only"=FALSE, "Identifier"="RSSCOPE_ATTR_SPECTRUM_ARITHMETIC_PARAMETER_MEASUREMENT_SPECTRUM", "Descriptive Name"="Spectrum Arithmetic Parameter Measurement Spectrum", "Data Type"=0, "Command"="MEAS{Measurement}:SPEC:ARIT:PAR{ArithmeticParameter}:SPEC", "Access"=2, "Range Table"="RsScope_rngSpectrumArithmeticMeasurementSpectrum", "Read Callback"="", "Write Callback"="", "Supported Models"="", "Instrument Options"="", "Flags"=0, "Help"="Selects the first operand for the sepctrum arithmetics measurements.\n\nAvailable Repeated Capabilities:\nMeasurement: Meas1, Meas2, Meas3, Meas4, Meas5, Meas6, Meas7, Meas8, Meas9, Meas10\r\nArithmeticParameter: ArithmeticParm1, ArithmeticParm2\r\n\nRemote-control command(s):\nMEASurement<m>:SPECtrum:ARIThmetic:PARameter<n>:SPECtrum"}, {"Level"=4, "Class Only"=FALSE, "Identifier"="RSSCOPE_ATTR_SPECTRUM_ARITHMETIC_OPERATOR", "Descriptive Name"="Spectrum Arithmetic Operator", "Data Type"=0, "Command"="MEAS{Measurement}:SPEC:ARIT:OPER", "Access"=2, "Range Table"="RsScope_rngSpectrumArithmeticOperator", 
